vi "Main.vi"   [LabVIEW 2017]
doc: "The start-up VI for our application and the UI"
uses:
  View Model/Controls/IO Type.ctl
types:
  T1 = typedef "View Model.ctl" = cluster{"Config Model":T2, "Error Model":T3, "Shared Model":T4, "Elevator Model":T5}
  T2 = typedef "Config Model.ctl" = cluster{"Config Change":refnum<user-event>, "Config Data":refnum<data-value>}
  T3 = typedef "Error Model.ctl" = cluster{"Error Event":refnum<user-event>}
  T4 = typedef "Shared Model.ctl" = cluster{"Stop Event":refnum<user-event>, "Stop DVR":refnum<data-value>}
  T5 = typedef "Elevator Model.ctl" = cluster{"Motion Change":refnum<user-event>, "Direction Change":refnum<user-event>, "Door Position Change":refnum<user-event>, "Emergency Change":refnum<user-event>, "Floor Change":refnum<user-event>, "Elevator CMD":refnum<user-event>, "Controller Overhead":refnum<data-value>}
  T6 = typedef "IO Type.ctl" = enum16{"Simulated", "Hardware"}
  T7 = enum32{"invalid app kind", "Development System", "Run Time System", "Student Edition", "Embedded LabVIEW", "Evaluation", "Custom"}
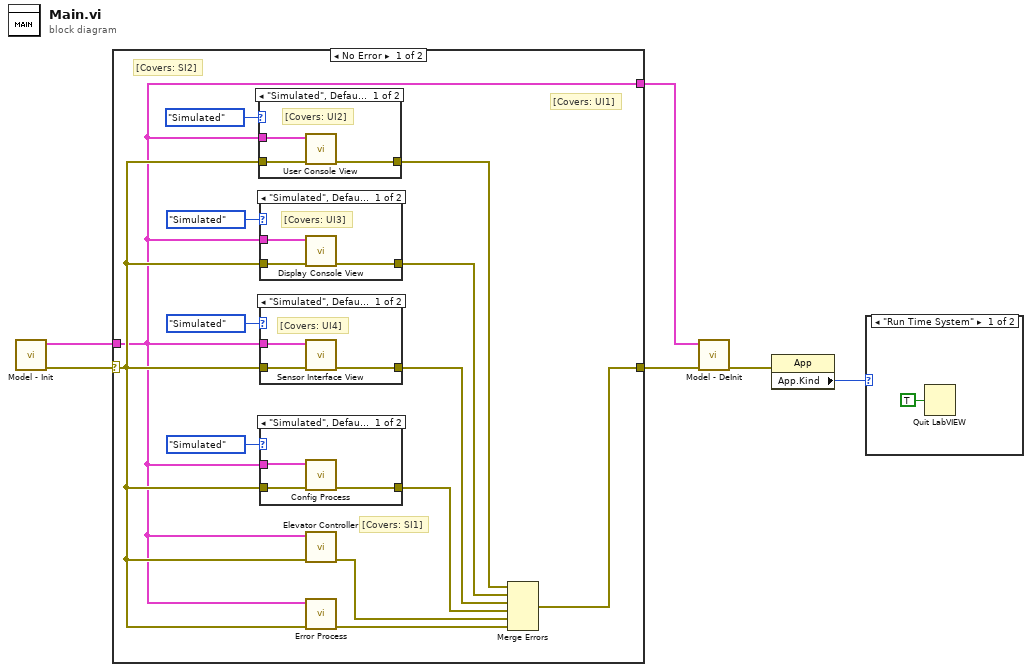
[diagram p0: block diagram]
diagram:
  n1 = call "Model - Init.vi"() -> ("error out"=w5:errorcluster, "View Model"=w6:T1)  [unwired: 10 in]
  n2 = case shown="No Error" w5 {
    selector: w5 -> [w9 w36]
    tunnel: w6 -> [w8 w37]
    tunnel: [w8 w37] -> w3
    tunnel: [w10 w36] -> w4
    frame No Error {
      # "[Covers: UI1]"
      # "[Covers: SI2]"
      # "[Covers: SI1]"
      n3 = case shown="\"Simulated\", Default" IO_Type."Simulated" ("Interface") {
        tunnel: w8 -> [w34 _]
        tunnel: w9 -> [w33 w35]
        tunnel: [w32 w35] -> w11
        frame "Simulated", Default {
          # "[Covers: UI2]"
          n4 = call "User Console View.vi"("error in (no error)"=w33, "View Model"=w34) -> ("error out"=w32:errorcluster)  [unwired: 9 in]
        }
        frame "Hardware" {
        }
      }
      n5 = case shown="\"Simulated\", Default" IO_Type."Simulated" ("Interface") {
        tunnel: w8 -> [w30 _]
        tunnel: w9 -> [w29 w31]
        tunnel: [w28 w31] -> w12
        frame "Simulated", Default {
          # "[Covers: UI3]"
          n6 = call "Display Console View.vi"("error in (no error)"=w29, "View Model"=w30) -> ("error out"=w28:errorcluster)  [unwired: 9 in]
        }
        frame "Hardware" {
        }
      }
      n7 = case shown="\"Simulated\", Default" IO_Type."Simulated" ("Interface") {
        tunnel: w8 -> [w26 _]
        tunnel: w9 -> [w25 w27]
        tunnel: [w24 w27] -> w13
        frame "Simulated", Default {
          # "[Covers: UI4]"
          n8 = call "Sensor Interface View.vi"("error in (no error)"=w25, "View Model"=w26) -> ("error out"=w24:errorcluster)  [unwired: 8 in, 1 out]
        }
        frame "Hardware" {
        }
      }
      n9 = case shown="\"Simulated\", Default" IO_Type."Simulated" ("Interface") {
        tunnel: w8 -> [w20 _]
        tunnel: w9 -> [w22 w23]
        tunnel: [w21 w23] -> w14
        frame "Simulated", Default {
          n10 = call "Config Process.vi"("error in (no error)"=w22, "View Model"=w20) -> ("error out"=w21:errorcluster)  [unwired: 9 in]
        }
        frame "Hardware" {
          # "Embedded DB"
        }
      }
      n11 = call "Elevator Controller.vi"("error in (no error)"=w9, "View Model"=w8) -> ("error out"=w7:errorcluster)  [unwired: 9 in]
      n12 = call "Error Process.vi"("error in (no error)"=w9, "View Model"=w8) -> ("error out"=w15:errorcluster)  [unwired: 9 in]
      n13 = Merge Errors(w11, w12, w13, w14, w7, w15) -> (w10:errorcluster)
    }
    frame Error {
    }
  }
  n14 = call "Model - DeInit.vi"("error in (no error)"=w4, "View Model"=w3) -> ("error out"=w2:errorcluster)  [unwired: 9 in]
  n15 = property class="App"(error in=w2) -> ("App.Kind"=w1:T7)  [unwired: 1 in, 2 out]
  n16 = case shown="\"Run Time System\"" w1 {
    frame "Run Time System" {
      n17 = Quit LabVIEW(quit? (T)=TRUE) -> ()
    }
    frame "Development System", Default {
    }
  }
